vi "Get TX Message.vi"(8 "error in (no error)":errorcluster, 11 "RxTx in":refnum<class "RxTx.lvclass">) -> (0 "error out":errorcluster, 2 "New msg":bool, 3 "RxTx out":refnum<class "RxTx.lvclass">)   [LabVIEW 2018, in "RxTx.lvclass"]
doc: "Pop the lastest Tx message found in the qeue"
uses:
  RxTx.lvclass
  RxTx.lvclass/RxTx.ctl
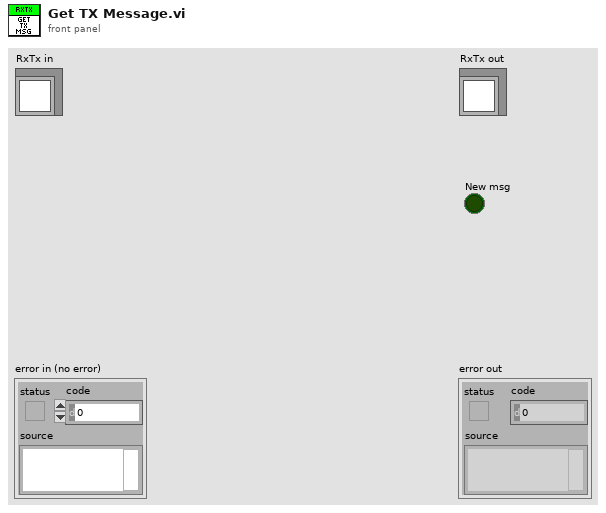
[diagram p1: front panel]
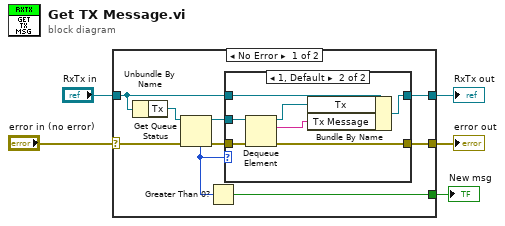
[diagram p0: block diagram]
diagram:
  n1 = case shown="No Error" "error in (no error)" {
    selector: "error in (no error)" -> [w11 w25]
    tunnel: [w9 w25] -> w3
    tunnel: [w13 w24] -> w2
    tunnel: "RxTx in" -> [w14 w24]
    tunnel: [w6 _] -> w1
    frame No Error {
      n2 = Unbundle By Name(w14) -> ("Tx"=w12:refnum<queue>)
      n3 = Get Queue Status(queue=w12, error in (no error)=w11) -> (queue out=w8:refnum<queue>, error out=w10:errorcluster, # elements in queue=w7:i32)  [unwired: 1 in, 5 out]
      n4 = Greater Than 0?(x=w7) -> (x > 0?=w6:bool)
      n5 = case shown="1, Default" w7 {
        tunnel: w14 -> [w15 w23]
        tunnel: [w15 w22] -> w13
        tunnel: w10 -> [w16 w20]
        tunnel: [w16 w19] -> w9
        tunnel: w8 -> [_ w18]
        frame 0 {
        }
        frame 1, Default {
          n6 = Dequeue Element(queue=w18, error in (no error)=w20) -> (queue out=w17:refnum<queue>, element=w21:string, error out=w19:errorcluster)  [unwired: 1 in, 1 out]
          n7 = Bundle By Name(cluster=w23, "Tx"=w17, "Tx Message"=w21) -> (w22:refnum<class "RxTx.lvclass">)
        }
      }
    }
    frame Error {
    }
  }
  "error out" <- w3
  "RxTx out" <- w2
  "New msg" <- w1
